vi "DetectAndKillTeraterm.vi"(6 "CheckTeraTerm(T)":bool, 8 "error in (no error)":errorcluster) -> (0 "error out":errorcluster)   [LabVIEW 2018]
panel:
  out "tterm running?(t)":bool
  out "standard output":string
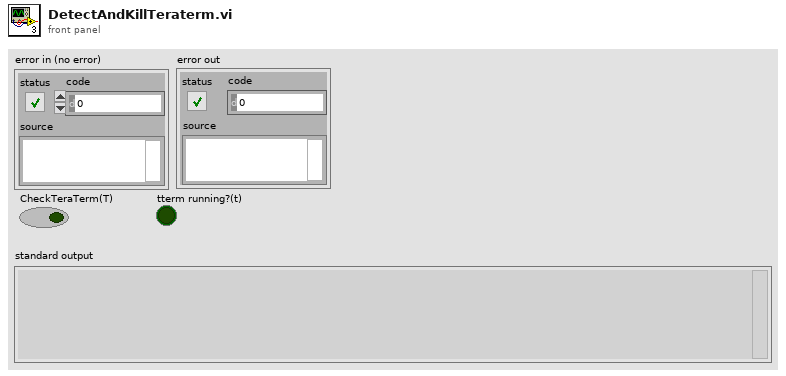
[diagram p1: front panel]
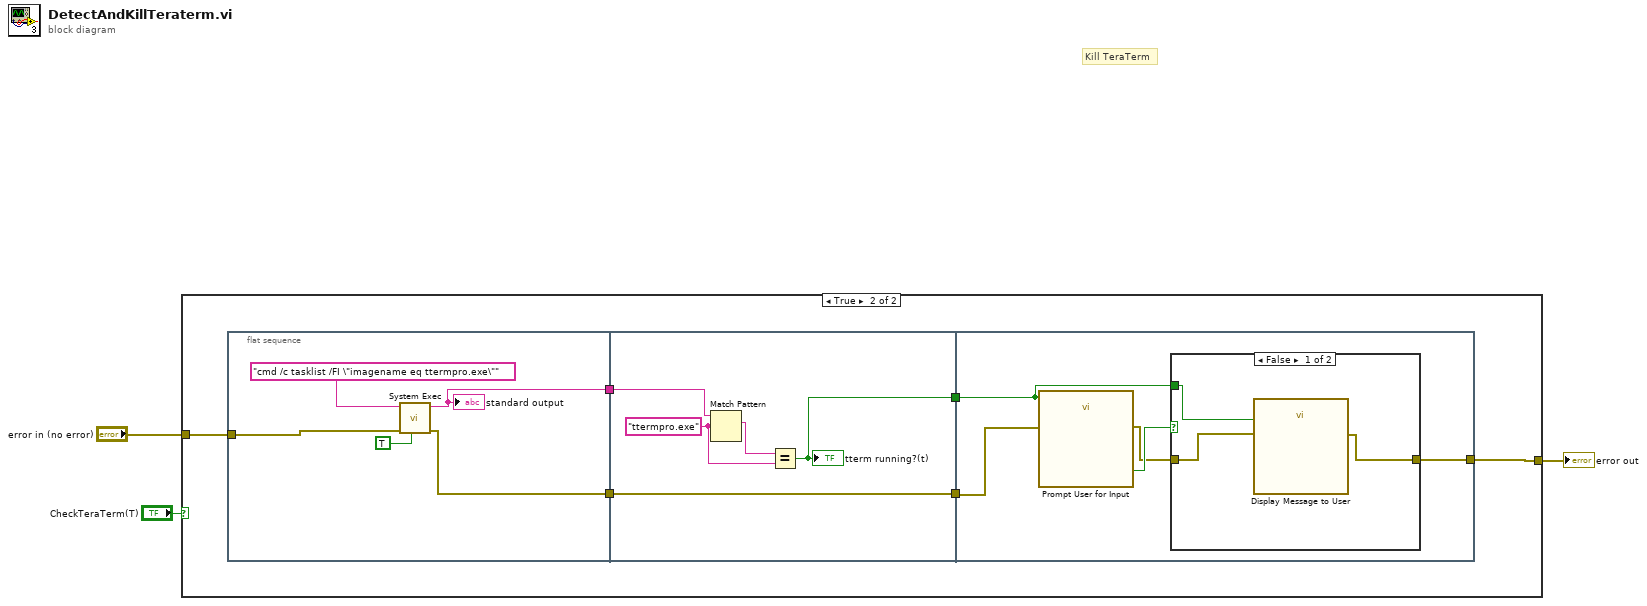
[diagram p0: block diagram]
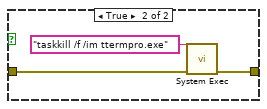
[diagram p3: hidden frame]
diagram:
  # "Kill TeraTerm"
  n1 = case shown="True" "CheckTeraTerm(T)" {
    tunnel: "error in (no error)" -> [w4 w6]
    tunnel: [w4 w5] -> w2
    frame False {
    }
    frame True {
      n2 = flat-sequence {
        tunnel: w6 -> [w13]
        tunnel: [w12] -> w10
        tunnel: [w11] -> w9
        tunnel: w10 -> [w20]
        tunnel: [w17] -> w8
        tunnel: [w16] -> w7
        tunnel: w9 -> [w16]
        tunnel: w8 -> [w21]
        tunnel: w7 -> [w24]
        tunnel: [w22] -> w5
        frame #0 {
          n3 = call <vilib>:"System Exec.vi"("run minimized? (F)"=TRUE, "error in (no error)"=w13, "command line"="cmd /c tasklist /FI \"imagename eq ttermpro.exe\"") -> ("error out"=w11:errorcluster, "standard output"=w12:string)  [unwired: 5 in, 2 out]
          "standard output" <- w12
        }
        frame #1 {
          w18 = "ttermpro.exe" ("regular expression")
          n4 = Match Pattern(string=w20, regular expression=w18) -> (match substring=w19:string)  [unwired: 1 in, 3 out]
          n5 = Equal?(x=w19, y=w18) -> (x = y?=w17:bool)
          "tterm running?(t)" <- w17
        }
        frame #2 {
          n6 = call "Prompt User for Input"("Enable"=w21, "error in (no error)"=w24) -> ("OK(Kill It)"=w25:bool, "error out"=w23:errorcluster)  [unwired: 16 in]
          n7 = case shown="False" w25 {
            tunnel: w23 -> [w28 w30]
            tunnel: [w27 w29] -> w22
            tunnel: w21 -> [w26 _]
            frame False {
              n8 = call "Display Message to User"("error in (no error)"=w28, "Enable"=w26) -> ("error out"=w27:errorcluster)  [unwired: 8 in, 1 out]
            }
            frame True {
              n9 = call <vilib>:"System Exec.vi"("error in (no error)"=w30, "command line"="taskkill /f /im ttermpro.exe") -> ("error out"=w29:errorcluster)  [unwired: 6 in, 3 out]
            }
          }
        }
      }
    }
  }
  "error out" <- w2
